vi "PC-Main.vi"() -> ()   [LabVIEW 2021]
panel:
  in  "Server":string="192.168.4.75"
  out "Output":bool[](array[boolean])
  out "Loop":i32
  in  "stop":bool
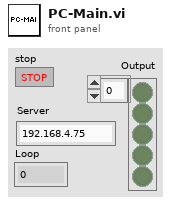
[diagram p1: front panel]
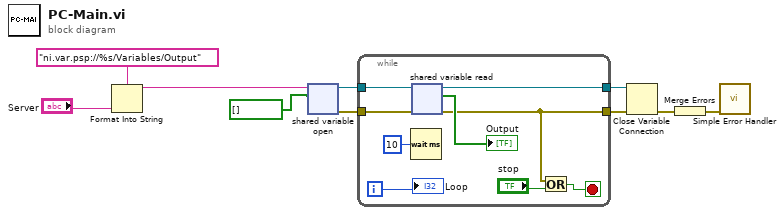
[diagram p0: block diagram]
diagram:
  n1 = Format Into String(format string="ni.var.psp://%s/Variables/Output", "Server") -> (resulting string=w2:string)  [unwired: 2 in, 1 out]
  n2 = shared-variable-open(w2, bool[] []) -> (w10:refnum<k21>, w5:errorcluster)  [unwired: 2 in]
  n3 = while {
    tunnel: w10 -> [w17]
    tunnel: [w12] -> w9
    tunnel: w5 -> [w15]
    tunnel: [w11] -> w4
    i -> [w18]
    stop <- w14 stop-if-true
    n4 = Wait (ms)(milliseconds to wait=u32 10) -> ()  [unwired: 1 out]
    n5 = shared-variable-read(w17, w15) -> (w12:refnum<k21>, w11:errorcluster, →"Output":bool[])  [unwired: 1 out]
    n6 = Or(x=w11, y="stop") -> (x .or. y?=w14:bool)
    "Loop" <- w18
  }
  n7 = Close Variable Connection(8:w4, 11:w9) -> (0:w8:errorcluster)
  n8 = Merge Errors(w8) -> (w7:errorcluster)
  n9 = call <vilib>:"Simple Error Handler.vi"("error in (no error)"=w7) -> ()  [unwired: 4 in, 5 out]
